vi "TEST_SUM&ADDS_(2ND).vi"(11 "Instrument VISA in":T1={"AWG VISA"="AgilentGenerator1", "Oscilloscope  VISA "="AgilentOsciloscope", "Integration Board IP"="172.16.17.47", "connection ID"=refnum, "report out"=refnum, "report file path"=path "C:/Documents and Settings/CTA_LAB01/Desktop/L0_Asic/L0 Asic Test Data"}) -> (0 "error out":errorcluster, 3 "Instrument VISA out":T1={"AWG VISA"="AgilentGenerator1", "Oscilloscope  VISA "="AgilentOsciloscope", "Integration Board IP"="172.16.17.47", "connection ID"=refnum, "report out"=refnum, "report file path"=path "C:/Documents and Settings/CTA_LAB01/Desktop/L0_Asic/L0 Asic Test Data"})   [LabVIEW 2012]
uses:
  <vilib>/Utility/NIReport.llb/NI_report.lvclass
  <vilib>/Utility/NIReport.llb/HTML/NI_HTML.lvclass
panel:
  in  "error in (no error)":errorcluster
  in  "stop":bool
  in  "Enable 6":bool=TRUE
  in  "Enable 4":bool=TRUE
  in  "Enable 5":bool=TRUE
  in  "Enable 2":bool=TRUE
  in  "Enable 3":bool=TRUE
  in  "Enable 0":bool=TRUE
  in  "Enable 1":bool=TRUE
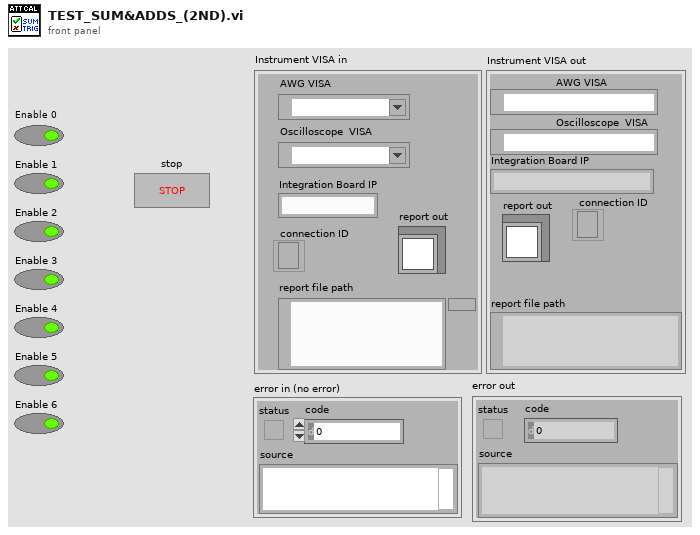
[diagram p1: front panel]
types:
  T1 = cluster{"AWG VISA":refnum<visa-resource-name>, "Oscilloscope  VISA ":refnum<visa-resource-name>, "Integration Board IP":string, "connection ID":refnum<k5>, "report out":refnum<class "NI_report.lvclass">, "report file path":path}
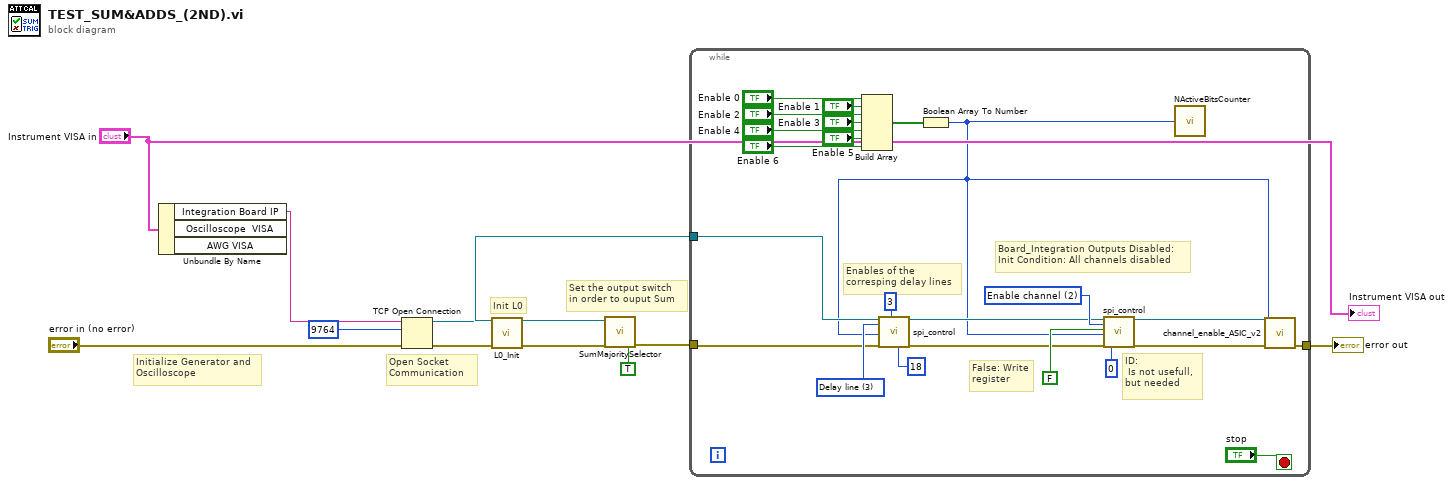
[diagram p0: block diagram]
diagram:
  # "Initialize Generator and \nOscilloscope"
  # "Init L0"
  # "Set the output switch\nin order to ouput Sum"
  # "Open Socket\nCommunication"
  n1 = Unbundle By Name("Instrument VISA in") -> ("Integration Board IP"=w8:string)  [unwired: 2 out]
  n2 = TCP Open Connection(address=w8, remote port or service name=u16 9764, error in (no error)="error in (no error)") -> (connection ID=w6:refnum<k5>, error out=w5:errorcluster)  [unwired: 2 in]
  n3 = call "L0_Init.vi"("error in"=w5, "connection ID in"=w6) -> ("error out"=w3:errorcluster, "connection ID out"=w4:refnum<k5>)  [unwired: 8 in]
  n4 = call "SumMajoritySelector.vi"("On Sum\nOff Majority"=TRUE ("On Sum\nOff Majority"), "error in (no error)"=w3, "connection ID"=w4) -> ("error out"=w2:errorcluster, "connection ID out"=w10:refnum<k5>)  [unwired: 5 in]
  n5 = while {
    tunnel: w10 -> [w35]
    tunnel: w2 -> [w14]
    tunnel: [w13] -> w9
    stop <- "stop" stop-if-true
    w30 = u16 2 items=["Attenuation", "Clipping", "Enable channel", "Delay line", "ASIC"] ("Device")
    w32 = u16 3 items=["Attenuation", "Clipping", "Enable channel", "Delay line", "ASIC"] ("Device")
    # "Enables of the\ncorresping delay lines"
    # "False: Write\nregister"
    # "ID:\n Is not usefull, \nbut needed"
    # "Board_Integration Outputs Disabled:\nInit Condition: All channels disabled"
    n6 = Build Array("Enable 0", "Enable 1", "Enable 2", "Enable 3", "Enable 4", "Enable 5", "Enable 6") -> (w24:bool[])
    n7 = Boolean Array To Number(Boolean array=w24) -> (number=w16:u32)
    n8 = call "spi_control.vi"("connection ID"=w35, "Device"=w32, "Data"=w16, "Register or channel"=18, "error in"=w14, "chip delay"=3) -> ("connection ID out"=w28:refnum<k5>, "error out 2"=w27:errorcluster)  [unwired: 6 in, 6 out]
    n9 = call "spi_control.vi"("connection ID"=w28, "Device"=w30, "Read/#write"=FALSE, "Data"=w16, "error in"=w27, "Id in"=0) -> ("connection ID out"=w26:refnum<k5>, "error out 2"=w25:errorcluster)  [unwired: 6 in, 6 out]
    n10 = call "NActiveBitsCounter.vi"("Input Number"=w16) -> ()  [unwired: 1 out]
    n11 = call "channel_enable_ASIC_v2.vi"("error in"=w25, "Channel Combination"=w16, "Connection ID in"=w26) -> ("error out"=w13:errorcluster)  [unwired: 7 in, 1 out]
  }
  "error out" <- w9
  "Instrument VISA out" <- "Instrument VISA in"
